vi "LidarParseDFA.vi"(10 "LIDAR raw data":u8) -> (0 "last measured value":u16, 1 "parser state":T1(ring), 2 "new value?":bool, 4 "angle":u8)   [LabVIEW 2010]
doc: "LidarParseDFA.vi parses the bytes returned by the LIDAR using a DFA to output data in range and scan angle.\n\n<b>Inputs</b>\nLIDAR raw data - the raw byte read in via serial from the LIDAR\n\n<b>Outputs</b>\nlast measured value - the last range value read in (in mm)\nangle - the angle of the last measured point\nparser state - the current state of the parser\ncm? - flags whether the LIDAR is returning data with cm instead mm resolution"
panel:
  out "cm?":u16
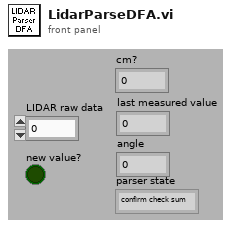
[diagram p1: front panel]
types:
  T1 = enum16{"confirm check sum", "check status byte", "read measured values", "confirm measurement", "confirm command", "read message length", "read address", "wait for \"02\""}
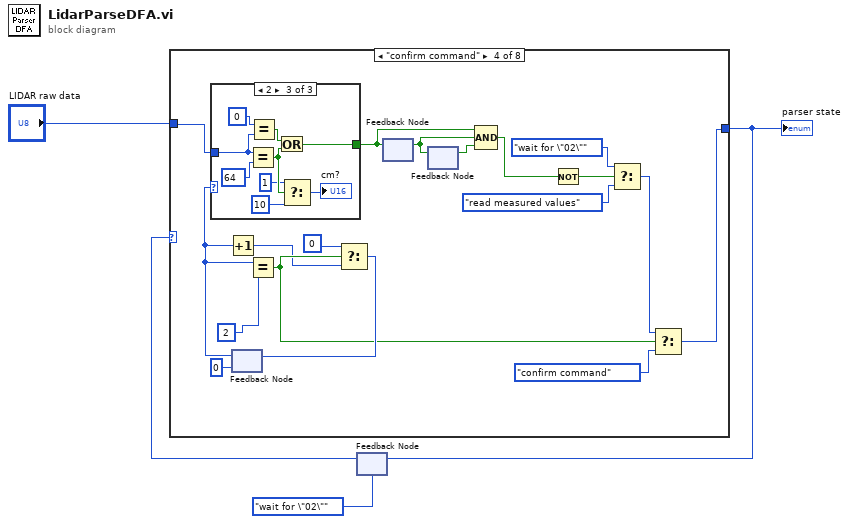
[diagram p0: block diagram]
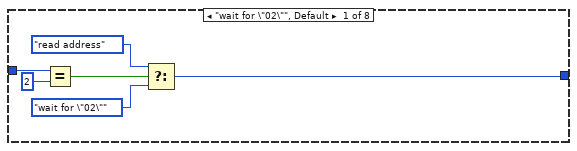
[diagram p2: hidden frame]
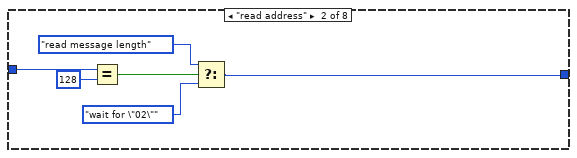
[diagram p3: hidden frame]
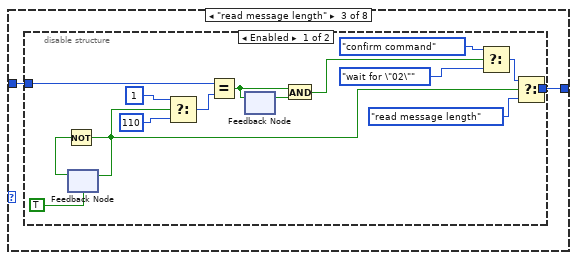
[diagram p4: hidden frame]
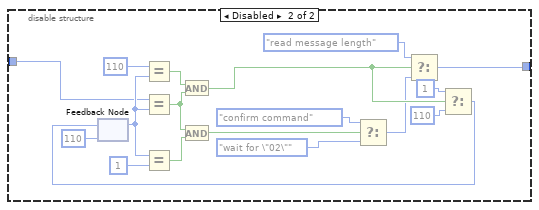
[diagram p5: hidden frame]
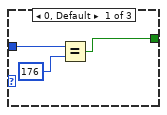
[diagram p6: hidden frame]
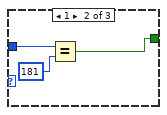
[diagram p7: hidden frame]
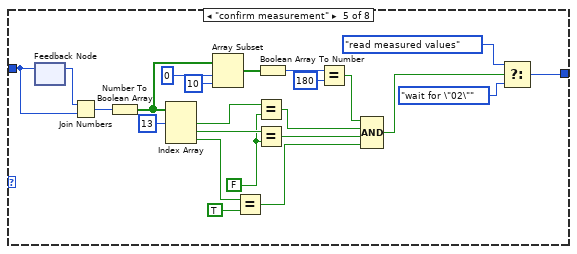
[diagram p8: hidden frame]
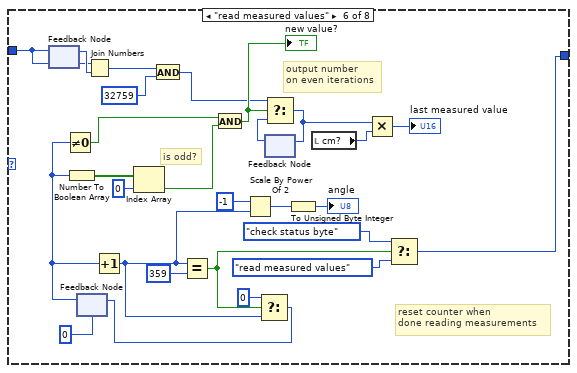
[diagram p9: hidden frame]
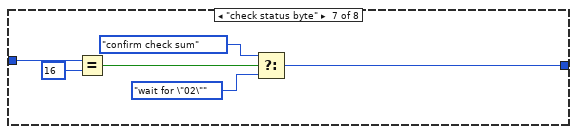
[diagram p10: hidden frame]
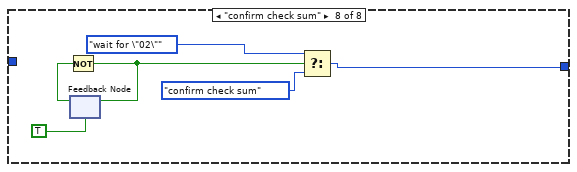
[diagram p11: hidden frame]
diagram:
  n1 = feedback #1(T1."wait for \"02\"") -> (w3:T1)
  n2 = case shown="\"confirm command\"" w3 {
    tunnel: "LIDAR raw data" -> [w10 w16 w17 w52 w106 w133 w140 _]
    tunnel: [w5 w11 w18 w57 w88 w118 w135 w141] -> w2
    frame "wait for \"02\"", Default {
      n3 = Equal?(x=w10, y=i8 2) -> (x = y?=w8:bool)
      n4 = Select(t=T1."read address", s=w8, f=T1."wait for \"02\"") -> (s? t:f=w5:T1)
    }
    frame "read address" {
      n5 = Equal?(x=w16, y=u8 128) -> (x = y?=w14:bool)
      n6 = Select(t=T1."read message length", s=w14, f=T1."wait for \"02\"") -> (s? t:f=w11:T1)
    }
    frame "read message length" {
      n7 = disable-structure shown="Enabled" {
        disable-tunnel: [w31 w35] -> w18
        disable-tunnel: w17 -> [w29 w34]
        frame Enabled {
          n8 = feedback #2(TRUE) -> (w33:bool)
          n9 = Not(x=w33) -> (.not. x?=w28:bool)
          n10 = feedback-in #2(w28) -> ()
          n11 = Select(t=u8 1 ("LIDAR raw data"), s=w28, f=u8 110 ("LIDAR raw data")) -> (s? t:f=w25:u8)
          n12 = Equal?(x=w29, y=w25) -> (x = y?=w20:bool)
          n13 = feedback #3() -> (w21:bool)  [unwired: 1 in]
          n14 = feedback-in #3(w20) -> ()
          n15 = And(x=w20, y=w21) -> (x .and. y?=w23:bool)
          n16 = Select(t=T1."confirm command", s=w23, f=T1."wait for \"02\"") -> (s? t:f=w19:T1)
          n17 = Select(t=w19, s=w28, f=T1."read message length") -> (s? t:f=w31:T1)
        }
        frame Disabled {
          n18 = feedback #4(u8 110 ("LIDAR raw data")) -> (w39:u8)
          n19 = Equal?(x=u8 110 ("LIDAR raw data"), y=w39) -> (x = y?=w37:bool)
          n20 = Equal?(x=w34, y=w39) -> (x = y?=w43:bool)
          n21 = Equal?(x=w39, y=u8 1 ("LIDAR raw data")) -> (x = y?=w42:bool)
          n22 = And(x=w37, y=w43) -> (x .and. y?=w48:bool)
          n23 = And(x=w43, y=w42) -> (x .and. y?=w46:bool)
          n24 = Select(t=T1."confirm command", s=w46, f=T1."wait for \"02\"") -> (s? t:f=w47:T1)
          n25 = Select(t=T1."read message length" ("f"), s=w48, f=w47) -> (s? t:f=w35:T1)
          n26 = Select(t=u8 1 ("LIDAR raw data"), s=w48, f=u8 110 ("LIDAR raw data")) -> (s? t:f=w51:u8)
          n27 = feedback-in #4(w51) -> ()
        }
      }
    }
    frame "confirm command" {
      n28 = feedback #5(u8 0 ("y")) -> (w54:u8)
      n29 = case shown="2" w54 {
        tunnel: w52 -> [w72 w75 w82]
        tunnel: [w70 w73 w80] -> w53
        frame 0, Default {
          n30 = Equal?(x=w72, y=u8 176) -> (x = y?=w70:bool)
        }
        frame 1 {
          n31 = Equal?(x=w75, y=u8 181) -> (x = y?=w73:bool)
        }
        frame 2 {
          n32 = Equal?(x=w82, y=u8 64) -> (x = y?=w79:bool)
          n33 = Equal?(x=u8 0 ("y"), y=w82) -> (x = y?=w81:bool)
          n34 = Or(x=w81, y=w79) -> (x .or. y?=w80:bool)
          n35 = Select(t=u16 1, s=w79, f=u16 10) -> (s? t:f=→"cm?":u16)
        }
      }
      n36 = Increment(x=w54) -> (x+1=w55:u8)
      n37 = Equal?(x=w54, y=u8 2) -> (x = y?=w60:bool)
      n38 = Select(t=u8 0 ("y"), s=w60, f=w55) -> (s? t:f=w67:u8)
      n39 = feedback-in #5(w67) -> ()
      n40 = feedback-in #6(w53) -> ()
      n41 = feedback #6() -> (w65:bool)  [unwired: 1 in]
      n42 = feedback-in #7(w65) -> ()
      n43 = feedback #7() -> (w64:bool)  [unwired: 1 in]
      n44 = Compound Arithmetic op=AND(w53, w65, w64) -> (w63:bool)
      n45 = Not(x=w63) -> (.not. x?=w62:bool)
      n46 = Select(t=T1."wait for \"02\"", s=w62, f=T1."read measured values") -> (s? t:f=w58:T1)
      n47 = Select(t=w58, s=w60, f=T1."confirm command") -> (s? t:f=w57:T1)
    }
    frame "confirm measurement" {
      w100 = FALSE ("y")
      n48 = feedback-in #8(w106) -> ()
      n49 = feedback #8() -> (w107:u8)  [unwired: 1 in]
      n50 = Join Numbers(hi=w107, lo=w106) -> ((hi.lo)=w105:u16)
      n51 = Number To Boolean Array(number=w105) -> (Boolean array=w95:bool[])
      n52 = Index Array(array=w95, index #1=13 ("index")) -> (element #1=w99:bool, element #2=w101:bool, element #3=w103:bool)  [unwired: 2 in]
      n53 = Array Subset(array=w95, index=0, length=10) -> (w92:bool[])
      n54 = Equal?(x=w103, y=TRUE) -> (x = y?=w96:bool)
      n55 = Equal?(x=w99, y=w100) -> (x = y?=w98:bool)
      n56 = Equal?(x=w101, y=w100) -> (x = y?=w97:bool)
      n57 = Boolean Array To Number(Boolean array=w92) -> (number=w91:u16)
      n58 = Equal?(x=w91, y=u16 180) -> (x = y?=w89:bool)
      n59 = Compound Arithmetic op=AND(w89, w98, w97, w96) -> (w87:bool)
      n60 = Select(t=T1."read measured values", s=w87, f=T1."wait for \"02\"") -> (s? t:f=w88:T1)
    }
    frame "read measured values" {
      # "is odd?"
      # "output number\non even iterations"
      # "reset counter when\ndone reading measurements"
      n61 = feedback-in #9(w133) -> ()
      n62 = feedback #9() -> (w134:u8)  [unwired: 1 in]
      n63 = feedback #10(i16 0) -> (w126:i16)
      n64 = Not Equal To 0?(x=w126) -> (x != 0?=w125:bool)
      n65 = Number To Boolean Array(number=w126) -> (Boolean array=w130:bool[])
      n66 = Join Numbers(hi=w133, lo=w134) -> ((hi.lo)=w115:u16)
      n67 = Increment(x=w126) -> (x+1=w113:i16)
      n68 = Index Array(array=w130, index=0) -> (element=w117:bool)
      n69 = And(x=w115, y=u16 32759) -> (x .and. y?=w114:u16)
      n70 = Equal?(x=w113, y=i16 359) -> (x = y?=w121:bool)
      n71 = And(x=w125, y=w117) -> (x .and. y?=w124:bool)
      "new value?" <- w124
      n72 = Scale By Power Of 2(n=-1, x=w113) -> (x*2^n=w111:i16)
      n73 = Select(t=i16 0, s=w121, f=w113) -> (s? t:f=w123:i16)
      n74 = feedback-in #10(w123) -> ()
      n75 = feedback #11() -> (w127:u16)  [unwired: 1 in]
      n76 = Select(t=w114, s=w124, f=w127) -> (s? t:f=w128:u16)
      n77 = feedback-in #11(w128) -> ()
      n78 = To Unsigned Byte Integer(number=w111) -> (unsigned 8bit integer=→"angle":u8)
      n79 = local read "cm?"() -> (w108:u16)
      n80 = Multiply(x=w128, y=w108) -> (x*y=→"last measured value":u16)
      n81 = Select(t=T1."check status byte", s=w121, f=T1."read measured values") -> (s? t:f=w118:T1)
    }
    frame "check status byte" {
      n82 = Equal?(x=w140, y=u8 16) -> (x = y?=w138:bool)
      n83 = Select(t=T1."confirm check sum", s=w138, f=T1."wait for \"02\"") -> (s? t:f=w135:T1)
    }
    frame "confirm check sum" {
      n84 = feedback #12(TRUE) -> (w146:bool)
      n85 = Not(x=w146) -> (.not. x?=w144:bool)
      n86 = feedback-in #12(w144) -> ()
      n87 = Select(t=T1."wait for \"02\"", s=w144, f=T1."confirm check sum") -> (s? t:f=w141:T1)
    }
  }
  "parser state" <- w2
  n88 = feedback-in #1(w2) -> ()
